vi "Flatten PDU1.vi"(8 "error in (no error)":errorcluster, 11 "Modbus data unit in":T1={"function"=1, "Data"=[]} {"function" items=["Read Discrete Inputs"=2, "Read Coils"=1, "Write Single Coil"=5, "Write Multiple Coils"=15, "Read Input Register"=4, "Read Holding Registers"=3, "Write Single Register"=6, "Write Multiple Registers"=16, "Read/Write Multiple Registers"=23, "Mask Write Register"=22, "Read FIFO Queue"=24, "Read File Record"=20, "Write File Record"=21, "Read Exception Status"=7, "Diagnostic"=8, "Get Com Event Counter"=11, "Get Com Event Log"=12, "Report Slave ID"=17, "Read Device Identification"=43]; "Data" format="%.0x"}) -> (0 "error out":errorcluster, 3 "full Modbus data unit":u8[](array[numeric]))   [LabVIEW 2019, in "NI_modbus_upd.lvlib"]
uses:
  NI_modbus_upd.lvlib
  Function.ctl
  Ctl/MB Modbus Data Unit.ctl
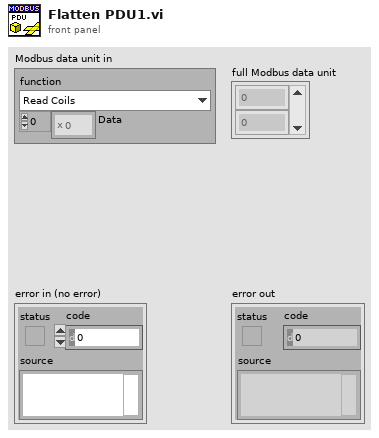
[diagram p1: front panel]
types:
  T1 = typedef "NI_modbus_upd.lvlib/MB Modbus Data Unit.ctl" = cluster{"function":T2, "Data":u8[]}
  T2 = typedef "NI_modbus_upd.lvlib/Function.ctl" = u8
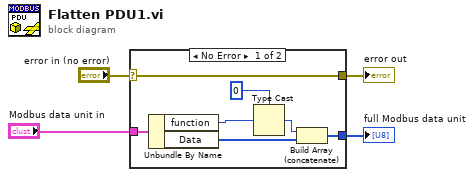
[diagram p0: block diagram]
diagram:
  n1 = case shown="No Error" "error in (no error)" {
    selector: "error in (no error)" -> [w5 w12]
    tunnel: "Modbus data unit in" -> [w11 _]
    tunnel: [w10 _] -> w3
    tunnel: [w5 w12] -> w1
    frame No Error {
      n2 = Unbundle By Name(w11) -> ("function"=w7:T2, "Data"=w6:u8[])
      n3 = Type Cast(type=u8 0, x=w7) -> (*(type *) &x=w9:u8)
      n4 = Build Array (concatenate)(w9, w6) -> (w10:u8[])
    }
    frame Error {
    }
  }
  "error out" <- w1
  "full Modbus data unit" <- w3
